vi "Configure Timing.vi"(8 "error in (no error)":errorcluster, 11 "Thermometer DAQmx Base CFG in":refnum<class "Thermometer DAQmx Base CFG.lvclass">) -> (0 "error out":errorcluster, 3 "Thermometer DAQmx Base CFG out":refnum<class "Thermometer DAQmx Base CFG.lvclass">)   [LabVIEW 2023, in "Thermometer DAQmx Base CFG.lvclass"]
uses:
  Thermometer DAQmx Base CFG.lvclass
  D:/git/HAL/HAL GOOP4/Configuration JSON Base/CFG JSON Base.lvclass
  Thermometer DAQmx Base CFG.lvclass/Thermometer DAQmx Base CFG.ctl
  3205de65-3c55-4af3-b1dc-a7065c343029.vi
  <vilib>/JDP Science/JSONtext/Find Item.vi
  <vilib>/JDP Science/JSONtext/Next JSON Value.vi
  <vilib>/JDP Science/JSONtext/String Subset.vi
  <vilib>/JDP Science/JSONtext/Parsing/Advance past next JSON Value (inlined COPY).vi
  <vilib>/JDP Science/JSONtext/Parsing/Advance past whitespace.vi
  <vilib>/JDP Science/JSONtext/Parsing/Advance past String.vi
  <vilib>/JDP Science/JSONtext/Parsing/Advance past Number.vi
  <vilib>/JDP Science/JSONtext/Parsing/Advance past Line Ending.vi
  <vilib>/JDP Science/JSONtext/Parsing/Parse Full Path or Item Name.vi
  <vilib>/JDP Science/JSONtext/Parsing/Advance past Array.vi
  <vilib>/JDP Science/JSONtext/Parsing/Advance past Object.vi
  <vilib>/JDP Science/JSONtext/support/Error Cluster From Code.vi
  <vilib>/JDP Science/JSONtext/Offset/Find Item Locations by Path.vi
  <vilib>/JDP Science/JSONtext/JSON text to Variant.vi
  <vilib>/Utility/error.llb/Error Cluster From Error Code.vi
  <vilib>/JDP Science/JSONtext/LVClass Serializer/JSONtext LVClass Serializer.lvclass
  <vilib>/ErrorRing/Error Ring.xnode
  <vilib>/DAQmx/configure/timing.llb/DAQmx Timing (Sample Clock).vi
  Configuration JSON Base/CFG JSON Base.lvclass
  D:/git/HAL/HAL GOOP4/Interfaces/IConfigure/IConfigure.lvclass
  D:/git/HAL/HAL GOOP4/Thermometer/Thermometer DAQmx Base CFG/Thermometer DAQmx Base CFG.lvclass
panel:
  out "Active Edge":i32(ring)=10280 items=["Rising"=10280, "Falling"=10171]
  out "Sample Mode":i32(ring)=10178 items=["Finite Samples"=10178, "Continuous Samples"=10123, "Hardware Timed Single Point"=12522]
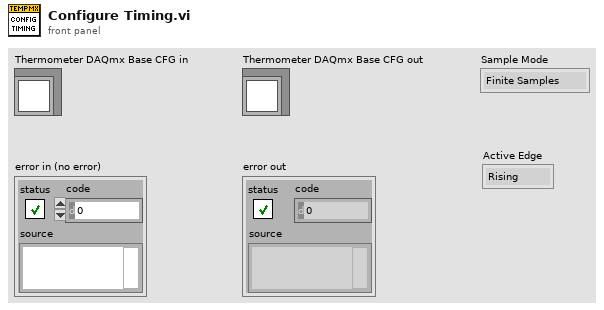
[diagram p1: front panel]
types:
  T1 = cluster{"Samples per Channel":i32, "Sample Mode":string, "Sample Rate":dbl, "Sample Clock Source":string, "Active Edge":string}
  T2 = typedef "LVStringsAndValuesArrayTypeDef_I32.ctl" = cluster{"String":string, "Value":i32}[]
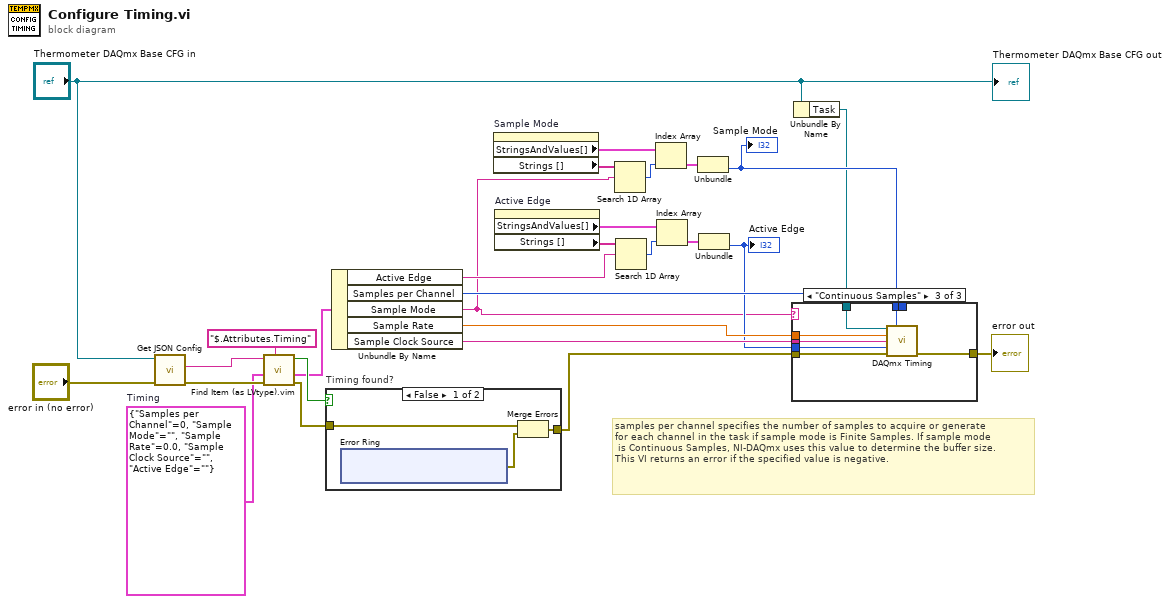
[diagram p0: block diagram]
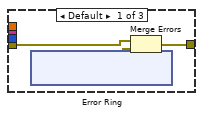
[diagram p2: hidden frame]
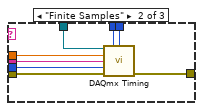
[diagram p3: hidden frame]
diagram:
  w23 = T1 {"Samples per Channel"=0, "Sample Mode"="", "Sample Rate"=0.0, "Sample Clock Source"="", "Active Edge"=""}  # Timing
  # "samples per channel specifies the number of samples to acquire or generate\nfor each channel in the task if sample mode is Finite Samples. If sample mode\n is Continuous Samples, NI-DAQmx uses this value to determine the buffer size.\nThis VI returns an error if the specified value is negative."
  n1 = call "Get JSON Config.vi"("error in (no error)"="error in (no error)", "CFG Base in"="Thermometer DAQmx Base CFG in") -> ("error out"=w27:errorcluster, "<JSON>Config>"=w26:string)  [unwired: 7 in, 1 out]
  n2 = call "Find Item (as LVtype).vim"("$Path or Item Name"="$.Attributes.Timing", "error in (no error)"=w27, "Data Type and Default Value"=w23, "JSON"=w26) -> ("error out"=w21:errorcluster, "Data"=w16:T1, "Found"=w22:bool)  [unwired: 4 in, 1 out]
  n3 = case "Timing found?" shown="False" w22 {
    tunnel: w21 -> [w29 w36]
    tunnel: [w28 w36] -> w15
    frame False {
      n4 = xnode "Error Ring"() -> ("error out"=w30:errorcluster)
      n5 = Merge Errors(w29, w30) -> (w28:errorcluster)
    }
    frame True {
    }
  }
  n6 = Unbundle By Name(w16) -> ("Active Edge"=w2:string, "Samples per Channel"=w7:i32, "Sample Mode"=w1:string, "Sample Rate"=w9:dbl, "Sample Clock Source"=w14:string)
  n7 = property on="Sample Mode" class="Ring (strict)"() -> ("StringsAndValues[]"=w18:T2, "Strings []"=w17:string[])  [unwired: 2 in, 2 out]
  n8 = property on="Active Edge" class="Ring (strict)"() -> ("StringsAndValues[]"=w12:T2, "Strings []"=w13:string[])  [unwired: 2 in, 2 out]
  n9 = Search 1D Array(1D array=w17, element=w1) -> (index of element=w19:i32)  [unwired: 1 in]
  n10 = Search 1D Array(1D array=w13, element=w2) -> (index of element=w11:i32)  [unwired: 1 in]
  n11 = Index Array(array=w18, index=w19) -> (element=w20:cluster{"String":string, "Value":i32})
  n12 = Index Array(array=w12, index=w11) -> (element=w10:cluster{"String":string, "Value":i32})
  n13 = Unbundle(w20) -> ("Value"=w8:i32)  [unwired: 1 out]
  "Sample Mode" <- w8
  n14 = Unbundle(w10) -> ("Value"=w3:i32)  [unwired: 1 out]
  "Active Edge" <- w3
  n15 = Unbundle By Name("Thermometer DAQmx Base CFG in") -> ("Task"=w6:refnum<k21>)
  n16 = case shown="\"Continuous Samples\"" w1 {
    tunnel: w15 -> [w38 w52 w59]
    tunnel: w14 -> [_ w51 w58]
    tunnel: w9 -> [_ w50 w57]
    tunnel: w8 -> [_ w49 w56]
    tunnel: w7 -> [_ w48 _]
    tunnel: w6 -> [_ w47 w55]
    tunnel: [w39 w46 w54] -> w4
    tunnel: w3 -> [_ w45 w53]
    frame Default {
      n17 = xnode "Error Ring"() -> ("error out"=w37:errorcluster)
      n18 = Merge Errors(w38, w37) -> (w39:errorcluster)
    }
    frame "Finite Samples" {
      n19 = call-poly <vilib>:"DAQmx Timing.vi"("task/channels in"=w47, "sample mode"=w49, "samples per channel"=w48, "rate"=w50, "source"=w51, "active edge"=w45, "error in"=w52) -> ("error out"=w46:errorcluster)  [unwired: 7 in, 1 out]
    }
    frame "Continuous Samples" {
      n20 = call-poly <vilib>:"DAQmx Timing.vi"("task/channels in"=w55, "sample mode"=w56, "rate"=w57, "source"=w58, "active edge"=w53, "error in"=w59) -> ("error out"=w54:errorcluster)  [unwired: 8 in, 1 out]
    }
  }
  "error out" <- w4
  "Thermometer DAQmx Base CFG out" <- "Thermometer DAQmx Base CFG in"
